vi "zmq_send.vi"(0 "error in":errorcluster, 2 "data":string, 3 "socket in":refnum<class "zmq_socket.lvclass">, 4 "more? (F)":bool) -> (5 "error out":errorcluster, 8 "socket out":refnum<class "zmq_socket.lvclass">)   [LabVIEW 2010, in "zeromq.lvlib" / "zmq_socket.lvclass"]
doc: "Add the binary string <b>data</b> (the NULL value \\0 is permitted) to the output queue of the socket <b>socket in</b>.\n\nIf <b>no block?</b> is True, the function returns immediately regardless of whether the message entered the queue successfully (not recommended).\n\nIf this message is part of a larger multi-component message and there are more parts to follow, then set <b>more?</b> to True.\n\nNote that when this call returns the message will likely <b>not have been sent yet</b> as it has only been placed in the queue for sending.\n\nDetailed API documentation: http://api.zeromq.org/3-2:zmq-send"
uses:
  zmq_socket.lvclass
  zmq_socket.lvclass/zmq_socket.ctl
  <vilib>/Utility/error.llb/Error Cluster From Error Code.vi
  zeromq.lvlib
panel:
  # "ØMQ"
  # "labview"
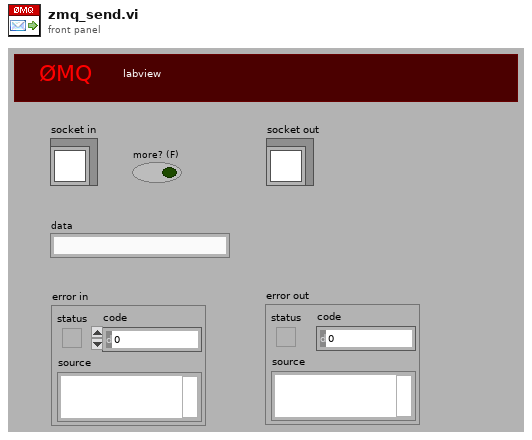
[diagram p1: front panel]
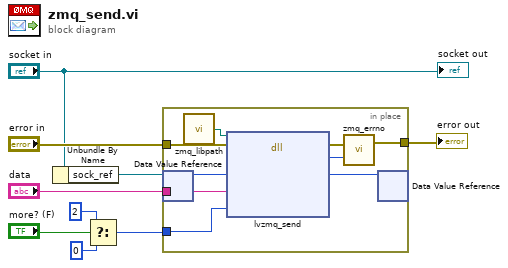
[diagram p0: block diagram]
diagram:
  n1 = Unbundle By Name("socket in") -> ("sock_ref"=w1:refnum<data-value>)
  n2 = Select(t=2 ("flags"), s="more? (F)", f=0 ("flags")) -> (s? t:f=w3:i32)
  n3 = in-place {
    in-place-border: "error in" -> [w18]
    in-place-border: "data" -> [w17]
    in-place-border: [w14] -> w7
    in-place-border: w3 -> [w13]
    n4 = in-place-dvr #1(w1) -> (w12:u64)  [unwired: 1 out]
    n5 = call "zmq_libpath.vi"() -> ("path"=w10:path)
    n6 = dll-call lib="?" fn="lvzmq_send" ("zmq_labview.dll:lvzmq_socket")(path in=w10, error in=w18, "sock_obj"=w12, "data"=w17, "flags"=w13) -> (error out=w16:errorcluster, "return type"=w15:i32, "sock_obj"=w11:u64)  [unwired: 3 in, 1 out]
    n7 = call "zmq_errno.vi"("retval"=w15, "error in"=w16) -> ("error out"=w14:errorcluster)  [unwired: 1 out]
    n8 = in-place-dvr #1(w11) -> ()  [unwired: 2 out]
  }
  "error out" <- w7
  "socket out" <- "socket in"
